vi "Zero Crossing.vi"   [LabVIEW 2017, in "NI_AdvCtrl_nonlinear.lvlib"]
doc: "LabVIEW no longer supports this VI. You can obtain similar functionality by installing the LabVIEW Simulation Module.\n\nDetects zero crossings of the input signal. The user can choose from three different detectors, either, minus-plus, and plus-minus."
uses:
  <vilib>/addons/control/advanced/NI_AdvCtrl_nonlinear.lvlib
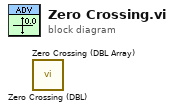
[diagram p0: block diagram]
diagram:
  n1 = call <vilib>:"Zero Crossing (DBL).vi"() -> ()  [unwired: 5 in, 1 out]
  n2 = call <vilib>:"Zero Crossing (DBL Array).vi"() -> ()  [unwired: 5 in, 1 out]
